vi "skipComment.vi"(8 "error in (no error)":errorcluster, 10 "Content":string[](array[string]), 11 "MatOper in":refnum<class "MatOper.lvclass">) -> (0 "error out":errorcluster, 2 "Modified Content":string[](array[string]), 3 "MatOper out":refnum<class "MatOper.lvclass">)   [LabVIEW 2016, in "OfcFunc.lvlib" / "MatOper.lvclass"]
doc: "Skip the comment (#) and empty line in the text array."
uses:
  MatOper.lvclass
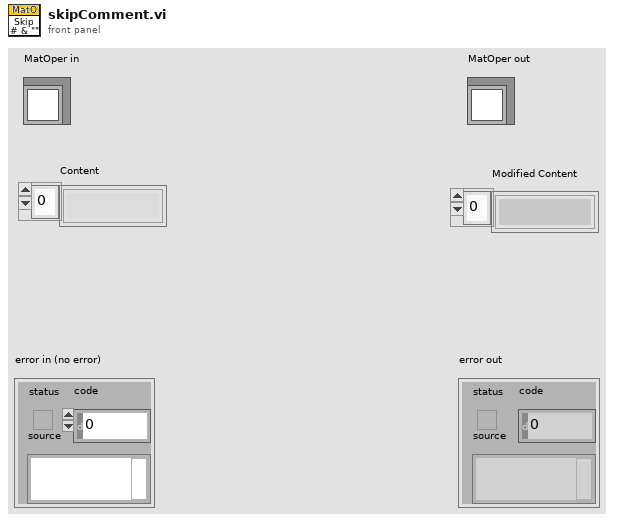
[diagram p1: front panel]
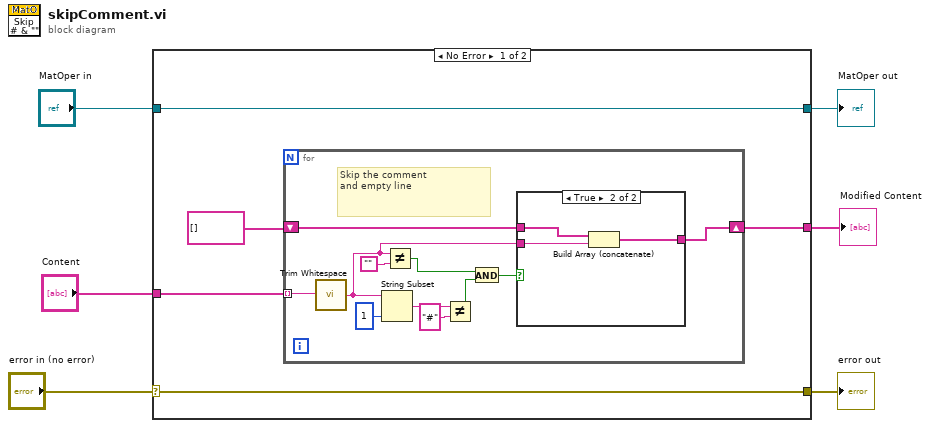
[diagram p0: block diagram]
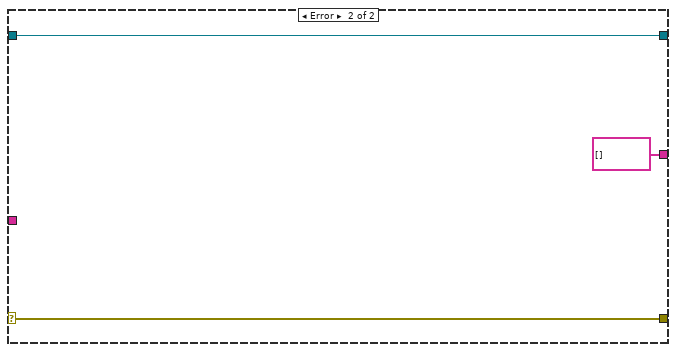
[diagram p3: hidden frame]
diagram:
  n1 = case shown="No Error" "error in (no error)" {
    selector: "error in (no error)" -> [w10 w29]
    tunnel: [w10 w29] -> w5
    tunnel: [w11 w28] -> w3
    tunnel: "MatOper in" -> [w11 w28]
    tunnel: [w8 string[] []] -> w2
    tunnel: "Content" -> [w7 _]
    frame No Error {
      n2 = for {
        tunnel: w7 -> [w18] mode=indexing
        shift-right: [w13] -> w8
        shift-left: string[] [] -> [w12]
        # "Skip the comment\nand empty line"
        n3 = call <vilib>:"Trim Whitespace.vi"("string"=w18) -> ("trimmed string"=w14:string)  [unwired: 1 in]
        n4 = String Subset(string=w14, length (rest)=1 ("length (rest)")) -> (substring=w21:string)  [unwired: 1 in]
        n5 = Not Equal?(x=w14, y="") -> (x != y?=w17:bool)
        n6 = Not Equal?(x=w21, y="#") -> (x != y?=w16:bool)
        n7 = And(x=w17, y=w16) -> (x .and. y?=w15:bool)
        n8 = case shown="True" w15 {
          tunnel: w14 -> [_ w26]
          tunnel: [w23 w25] -> w13
          tunnel: w12 -> [w23 w24]
          frame False {
          }
          frame True {
            n9 = Build Array (concatenate)(w24, w26) -> (w25:string[])
          }
        }
      }
    }
    frame Error {
    }
  }
  "error out" <- w5
  "MatOper out" <- w3
  "Modified Content" <- w2
